vi "OpenSession.vi"(8 "error in (no error)":errorcluster, 10 "gRPCid":T4, 11 "ctet_smu":T1) -> (0 "error out":errorcluster, 3 "ctet_smu out":T1)   [LabVIEW 2019, in "ctet_smu User Library.lvlib"]
uses:
  ctet_smu User Library.lvlib
  Servers/ctet_smu/gRPC lvSupport/Server API/typeDefs/grpcId.ctl
  Types/ctet_smu.ctl
  Servers/ctet_smu/ctet_smu Class/RPC Messages/measurementservice_SMUConfigResponse/measurementservice_SMUConfigResponse_Data.ctl
  Servers/ctet_smu/ctet_smu Class/RPC Messages/measurementservice_ErrorOut/measurementservice_ErrorOut_Data.ctl
  Servers/ctet_smu/ctet_smu Class/RPC Messages/measurementservice_SMUOpenSessionResponse/measurementservice_SMUOpenSessionResponse_Data.ctl
  Servers/ctet_smu/ctet_smu Class/ctet_smu.lvclass
  Servers/ctet_smu/gRPC lvSupport/gprc-lvsupport.lvlib
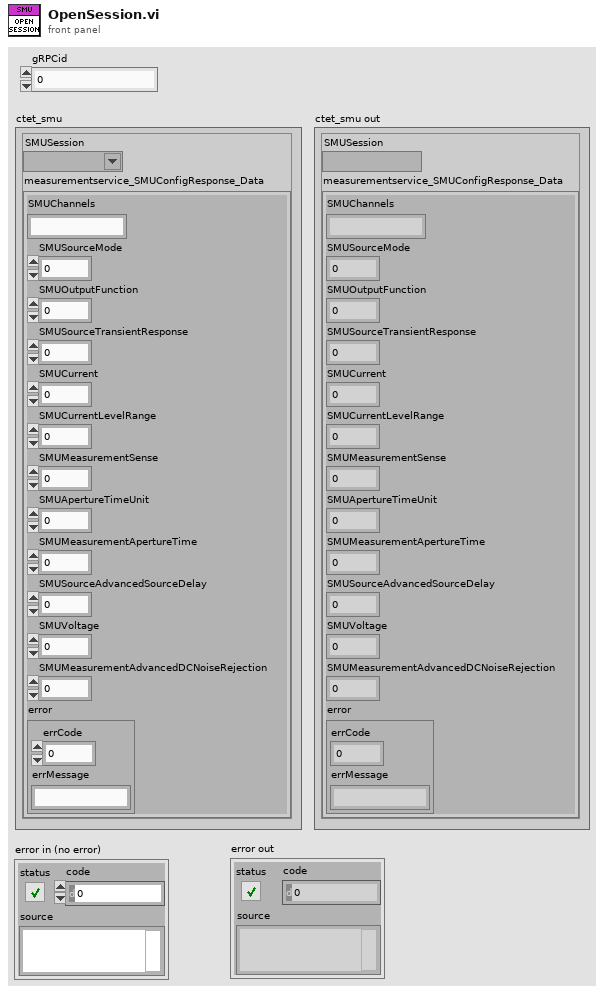
[diagram p1: front panel]
types:
  T1 = typedef "ctet_smu User Library.lvlib/ctet_smu.ctl" = cluster{"SMUSession":refnum<k15>, "measurementservice_SMUConfigResponse_Data":T2}
  T2 = typedef "ctet_smu.lvlib/ctet_smu.lvclass/measurementservice_SMUConfigResponse_Data.ctl" = cluster{"SMUChannels":string, "SMUSourceMode":i64, "SMUOutputFunction":i64, "SMUSourceTransientResponse":i64, "SMUCurrent":dbl, "SMUCurrentLevelRange":dbl, "SMUMeasurementSense":i64, "SMUApertureTimeUnit":i64, "SMUMeasurementApertureTime":dbl, "SMUSourceAdvancedSourceDelay":dbl, "SMUVoltage":dbl, "SMUMeasurementAdvancedDCNoiseRejection":i64, "error":T3}
  T3 = typedef "ctet_smu.lvlib/ctet_smu.lvclass/measurementservice_ErrorOut_Data.ctl" = cluster{"errCode":i64, "errMessage":string}
  T4 = typedef "ctet_smu.lvlib/gprc-lvsupport.lvlib/grpcId.ctl" = u64
  T5 = typedef "ctet_smu.lvlib/ctet_smu.lvclass/measurementservice_SMUOpenSessionResponse_Data.ctl" = cluster{"error":T3}
  T6 = typedef "ctet_smu.lvlib/ctet_smu.lvclass/measurementservice_SMUOpenSessionRequest_Data.ctl" = cluster{"SMUName":string, "SMUChannels":string}
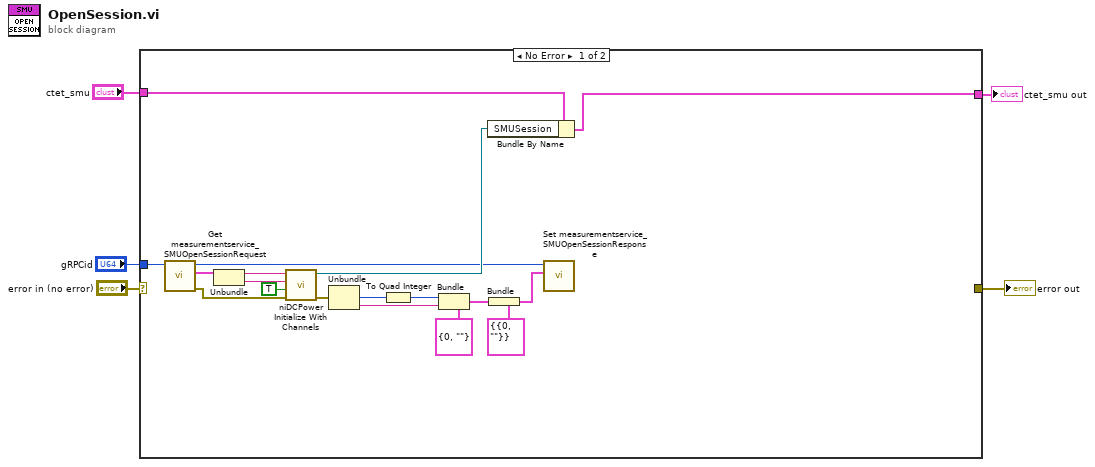
[diagram p0: block diagram]
diagram:
  n1 = case shown="No Error" "error in (no error)" {
    selector: "error in (no error)" -> [_ w25]
    tunnel: [_ w25] -> w5
    tunnel: "gRPCid" -> [w23 _]
    tunnel: "ctet_smu" -> [w17 w24]
    tunnel: [w15 w24] -> w1
    frame No Error {
      n2 = call "Get measurementservice_SMUOpenSessionRequest.vi"("gRPCid"=w23) -> ("error out"=w18:errorcluster, "Message Data"=w22:T6, "gRPCid out"=w13:T4)  [unwired: 8 in]
      n3 = Unbundle(w22) -> ("SMUName"=w20:string, "SMUChannels"=w21:string)
      n4 = call <instrlib>:"niDCPower Initialize With Channels.vi"("error in (no error)"=w18, "reset (false)"=TRUE, "channels"=w21, "resource name"=w20) -> ("error out"=w14:errorcluster, "instrument handle out"=w16:refnum<k15>)  [unwired: 6 in]
      n5 = Unbundle(w14) -> ("code"=w7:i32, "source"=w8:string)  [unwired: 1 out]
      n6 = To Quad Integer(1:w7) -> (0:w6:i64)
      n7 = Bundle(cluster=T3 {"errCode"=0, "errMessage"=""} ("error"), "errCode"=w6, "errMessage"=w8) -> (w9:T3)
      n8 = Bundle By Name(cluster=w17, "SMUSession"=w16) -> (w15:T1)
      n9 = Bundle(cluster=T5 {"error"={"errCode"=0, "errMessage"=""}} ("measurementservice_SMUOpenSessionResponse_Data"), "error"=w9) -> (w12:T5)
      n10 = call "Set measurementservice_SMUOpenSessionResponse.vi"("Message Data"=w12, "gRPCid"=w13) -> ()  [unwired: 9 in, 1 out]
    }
    frame Error {
    }
  }
  "error out" <- w5
  "ctet_smu out" <- w1
